vi "Servo_Button.vi"   [LabVIEW 2018]
uses:
  <vilib>/rvi/Emulation/niFpgaGetClockAttributes.vi
  <vilib>/rvi/Emulation/niFpgaSctlEmulationGetInTimedLoop.vi
  <vilib>/rvi/Emulation/niFpgaEmulationReportErrorSimple.vi
  <vilib>/rvi/eio/common/nirviEmuTemplateMethod_errors.vi
  <vilib>/rvi/Emulation/niFpgaCriticalErrorInLSC.vi
  <vilib>/eio/EIONode/EIONode.xnode
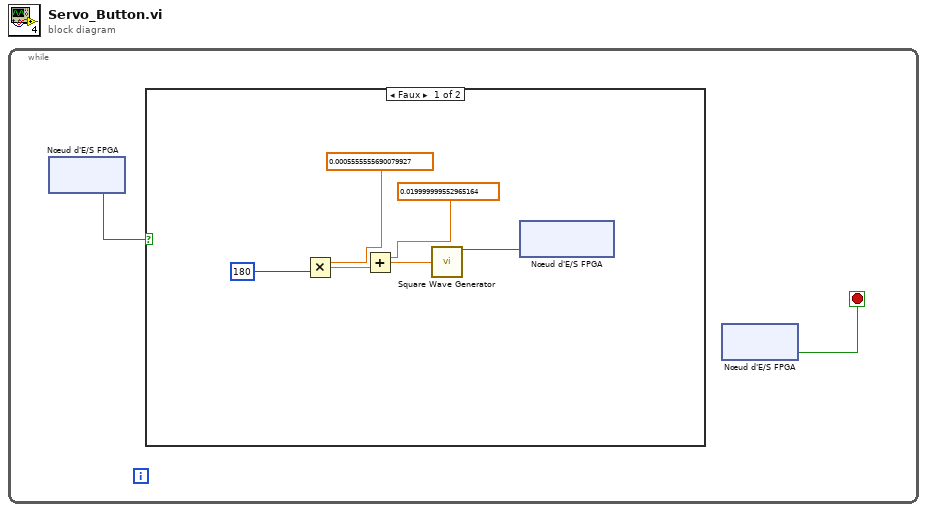
[diagram p0: block diagram]
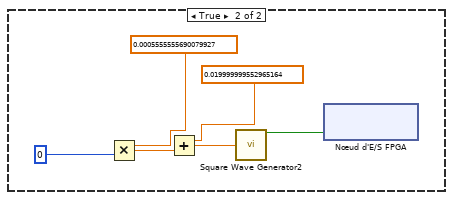
[diagram p2: hidden frame]
diagram:
  n1 = while {
    stop <- w2 stop-if-true
    n2 = xnode "Nœud d'E/S FPGA"() -> ("SW0"=w1:bool)  [unwired: 1 in, 1 out]
    n3 = case shown="Faux" w1 {
      frame False {
        n4 = Multiply(x=sgl 0.00055555557, y=i16 180) -> (x*y=w8:sgl)
        n5 = Add(x=sgl 0.02, y=w8) -> (x+y=w7:sgl)
        n6 = call "Square Wave Generator"("duty cycle (periods)"=w7) -> ("square wave out"=w6:bool)  [unwired: 14 in]
        n7 = xnode "Nœud d'E/S FPGA"("BB3_DIO0"=w6) -> ()  [unwired: 1 in, 1 out]
      }
      frame True {
        n8 = Multiply(x=sgl 0.00055555557, y=i16 0) -> (x*y=w14:sgl)
        n9 = Add(x=sgl 0.02, y=w14) -> (x+y=w13:sgl)
        n10 = call "Square Wave Generator2"("duty cycle (periods)"=w13) -> ("square wave out"=w12:bool)  [unwired: 14 in]
        n11 = xnode "Nœud d'E/S FPGA"("BB3_DIO0"=w12) -> ()  [unwired: 1 in, 1 out]
      }
    }
    n12 = xnode "Nœud d'E/S FPGA"() -> ("BTN0"=w2:bool)  [unwired: 1 in, 1 out]
  }
